vi "Sim_Control.vi"() -> ()   [LabVIEW 2009]
uses:
  <vilib>/addons/control/pid/pid.llb/PID (DBL).vi
  <vilib>/addons/control/pid/NI_PID_pid.lvlib
panel:
  out "desired turn rate and actual":cluster{"output":dbl, "Turn Rate Current":dbl}(graph)={"output"=0.0, "Turn Rate Current"=-0.0757104347794666}
  out "desired turn rate":dbl format="%.2f"
  in  "Overshoot Limit":dbl=10.0
  out "Turn Rate Current":dbl=2.609190335718722
  in  "stop":bool
  in  "Add 180":bool
  in  "Add 90":bool
  in  "Add 45":bool
  in  "Heading vs turn rate gains":T1={"proportional gain (Kc)"=-1.0, "integral time (Ti, min)"=0.0, "derivative time (Td, min)"=25.0} {"derivative time (Td, min)" format="%.5f"; "integral time (Ti, min)" format="%.5f"; "proportional gain (Kc)" format="%.5f"}
  in  "heading\ndeadband":dbl=2.0
  in  "Turn rate Control Loop":bool=TRUE
  out "Straight Voltages":cluster{"Left Voltage":dbl, "Right Voltage":dbl}
  out "Turning Voltages":cluster{"Left Voltage":dbl, "Right Voltage":dbl}={"Left Voltage"=2.5, "Right Voltage"=2.5}
  in  "Tab Control":enum32{"Sim", "Heading", "GPS"}(tab)=enum."Heading"
  out "XY Graph":T2(graph)
  out "Theta":dbl
  out "Display Heading":dbl
  in  "Initial Paremeters":T3
  out "Output Telemetry":T3
  out "Waveform Chart":T3(graph)
  in  "Iterations?":bool
  in  "Motor Voltages":cluster{"Left Voltage":dbl, "Right Voltage":dbl}={"Left Voltage"=5.0, "Right Voltage"=5.0}
  in  "Iterations":i32=300
  in  "Enable Step?":bool
  in  "step":bool
  out "Motors":cluster{"Left Voltage":dbl, "Right Voltage":dbl}(graph)
  out "Heading Error":cluster{dbl, "y":dbl, "y":dbl, "y":dbl}(graph)
  in  "Heading PID gains":T1={"proportional gain (Kc)"=0.2, "integral time (Ti, min)"=0.0, "derivative time (Td, min)"=10.0} {"derivative time (Td, min)" format="%.5f"; "integral time (Ti, min)" format="%.5f"; "proportional gain (Kc)" format="%.5f"}
  in  "Heading Control Loop?":bool=TRUE
  out "Compass Heading":dbl=1.0
  in  "Desired Heading":dbl
  out "Heading Chart":dbl(graph)
  in  "Compass Error (deg)":dbl=0.3
  in  "Compass Update Rate (hz)":dbl=8.0
  out "Longitude Chart":cluster{dbl, dbl, "Y":dbl}(graph)
  in  "GPS Update Rate (hz)":dbl=20.0
  in  "Latitude Error (m N)":dbl=1.3
  in  "Longitude Error (m E)":dbl=1.5
  out "Latitude":dbl=1.0
  out "Longitude":dbl=1.0
  out "Latitude Chart":cluster{dbl, dbl, "X":dbl}(graph)
  in  "Navigation Control Loop?":bool=TRUE
  out "Location Graph":T2(graph)
  in  "Deisired Latitude":dbl
  in  "Deisired Longitude":dbl
  out "distance to waypoint":dbl
  out "waypoint vector heading":dbl
  out "Averaged Latitude":dbl=1.0
  out "Averaged Longitude":dbl=1.0
  in  "GPS Averaging Samples":dbl=20.0
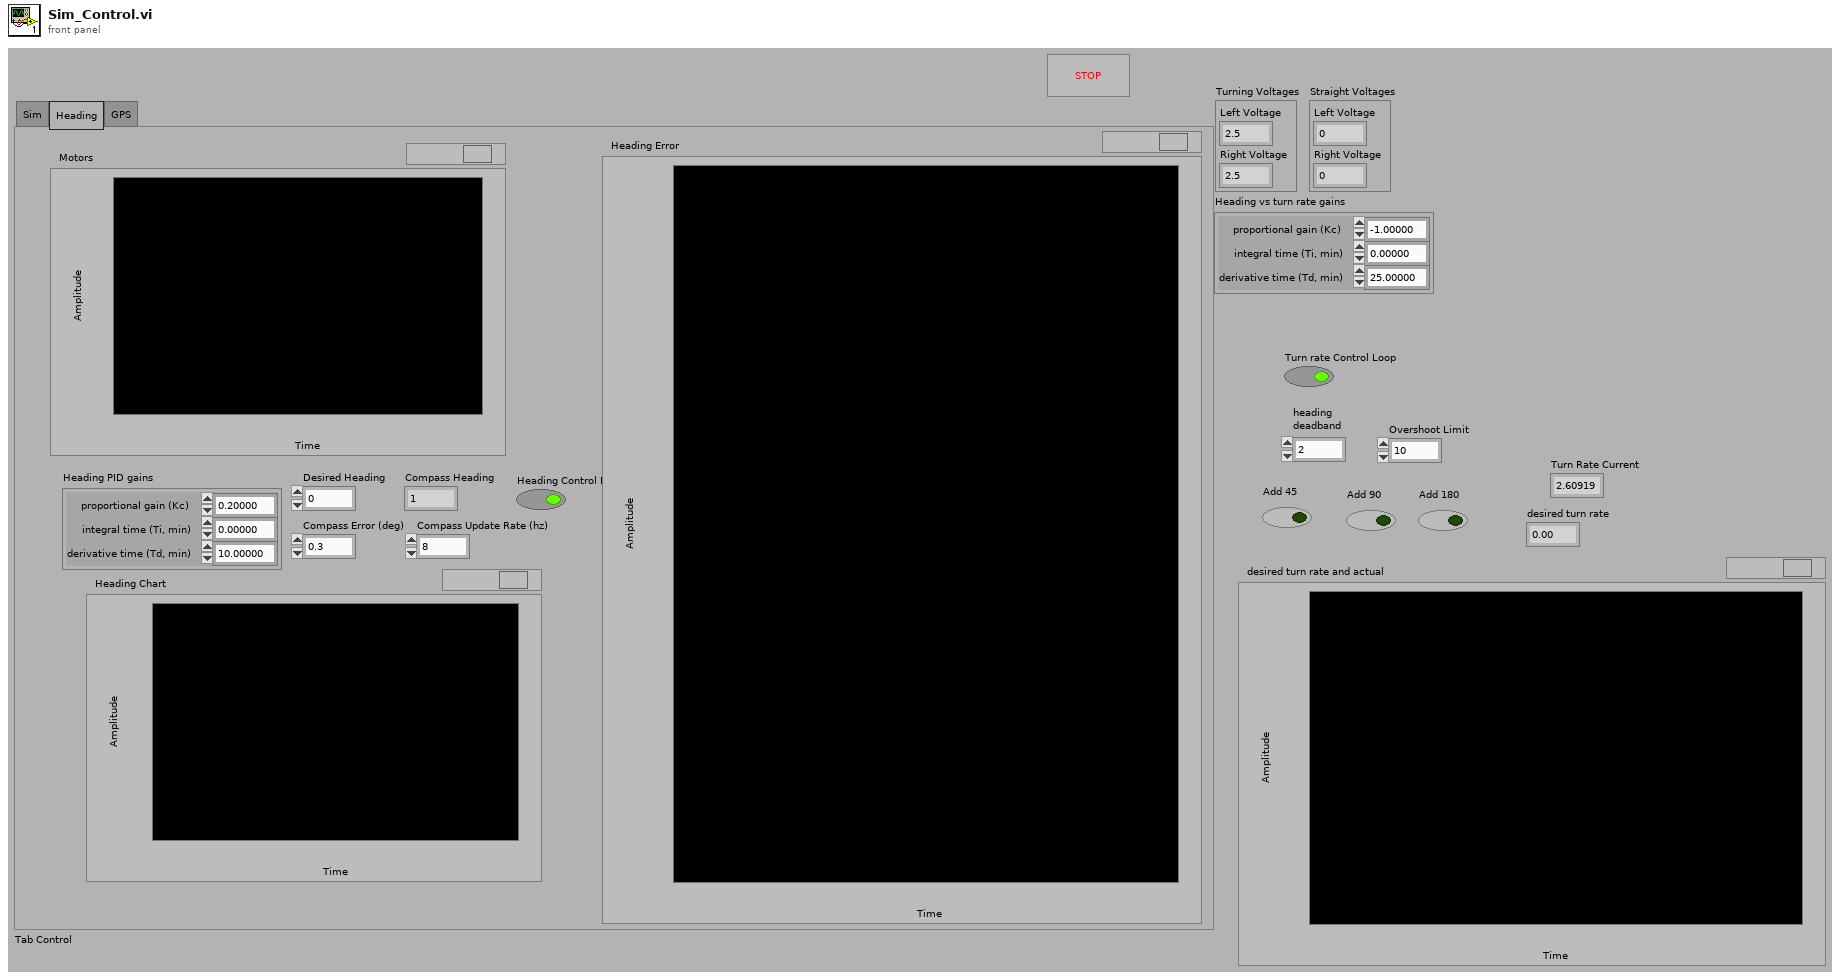
[diagram p1: front panel]
types:
  T1 = cluster{"proportional gain (Kc)":dbl, "integral time (Ti, min)":dbl, "derivative time (Td, min)":dbl}
  T2 = cluster{"initialized array":dbl[], "initialized array":dbl[]}[]
  T3 = cluster{"X":dbl, "Vx":dbl, "Ax":dbl, "Y":dbl, "Vy":dbl, "Ay":dbl, "Theta":dbl, "Omega":dbl, "Alpha":dbl}
  T4 = cluster{"X":dbl, "Vx":dbl, "Ax":dbl, "Y":dbl, "Vy":dbl, "Ay":dbl, "Theta":dbl, "Omega":dbl, "Alpha":dbl}[]
  T5 = cluster{dbl, "y":dbl, "Overshoot Limit":dbl, dbl}
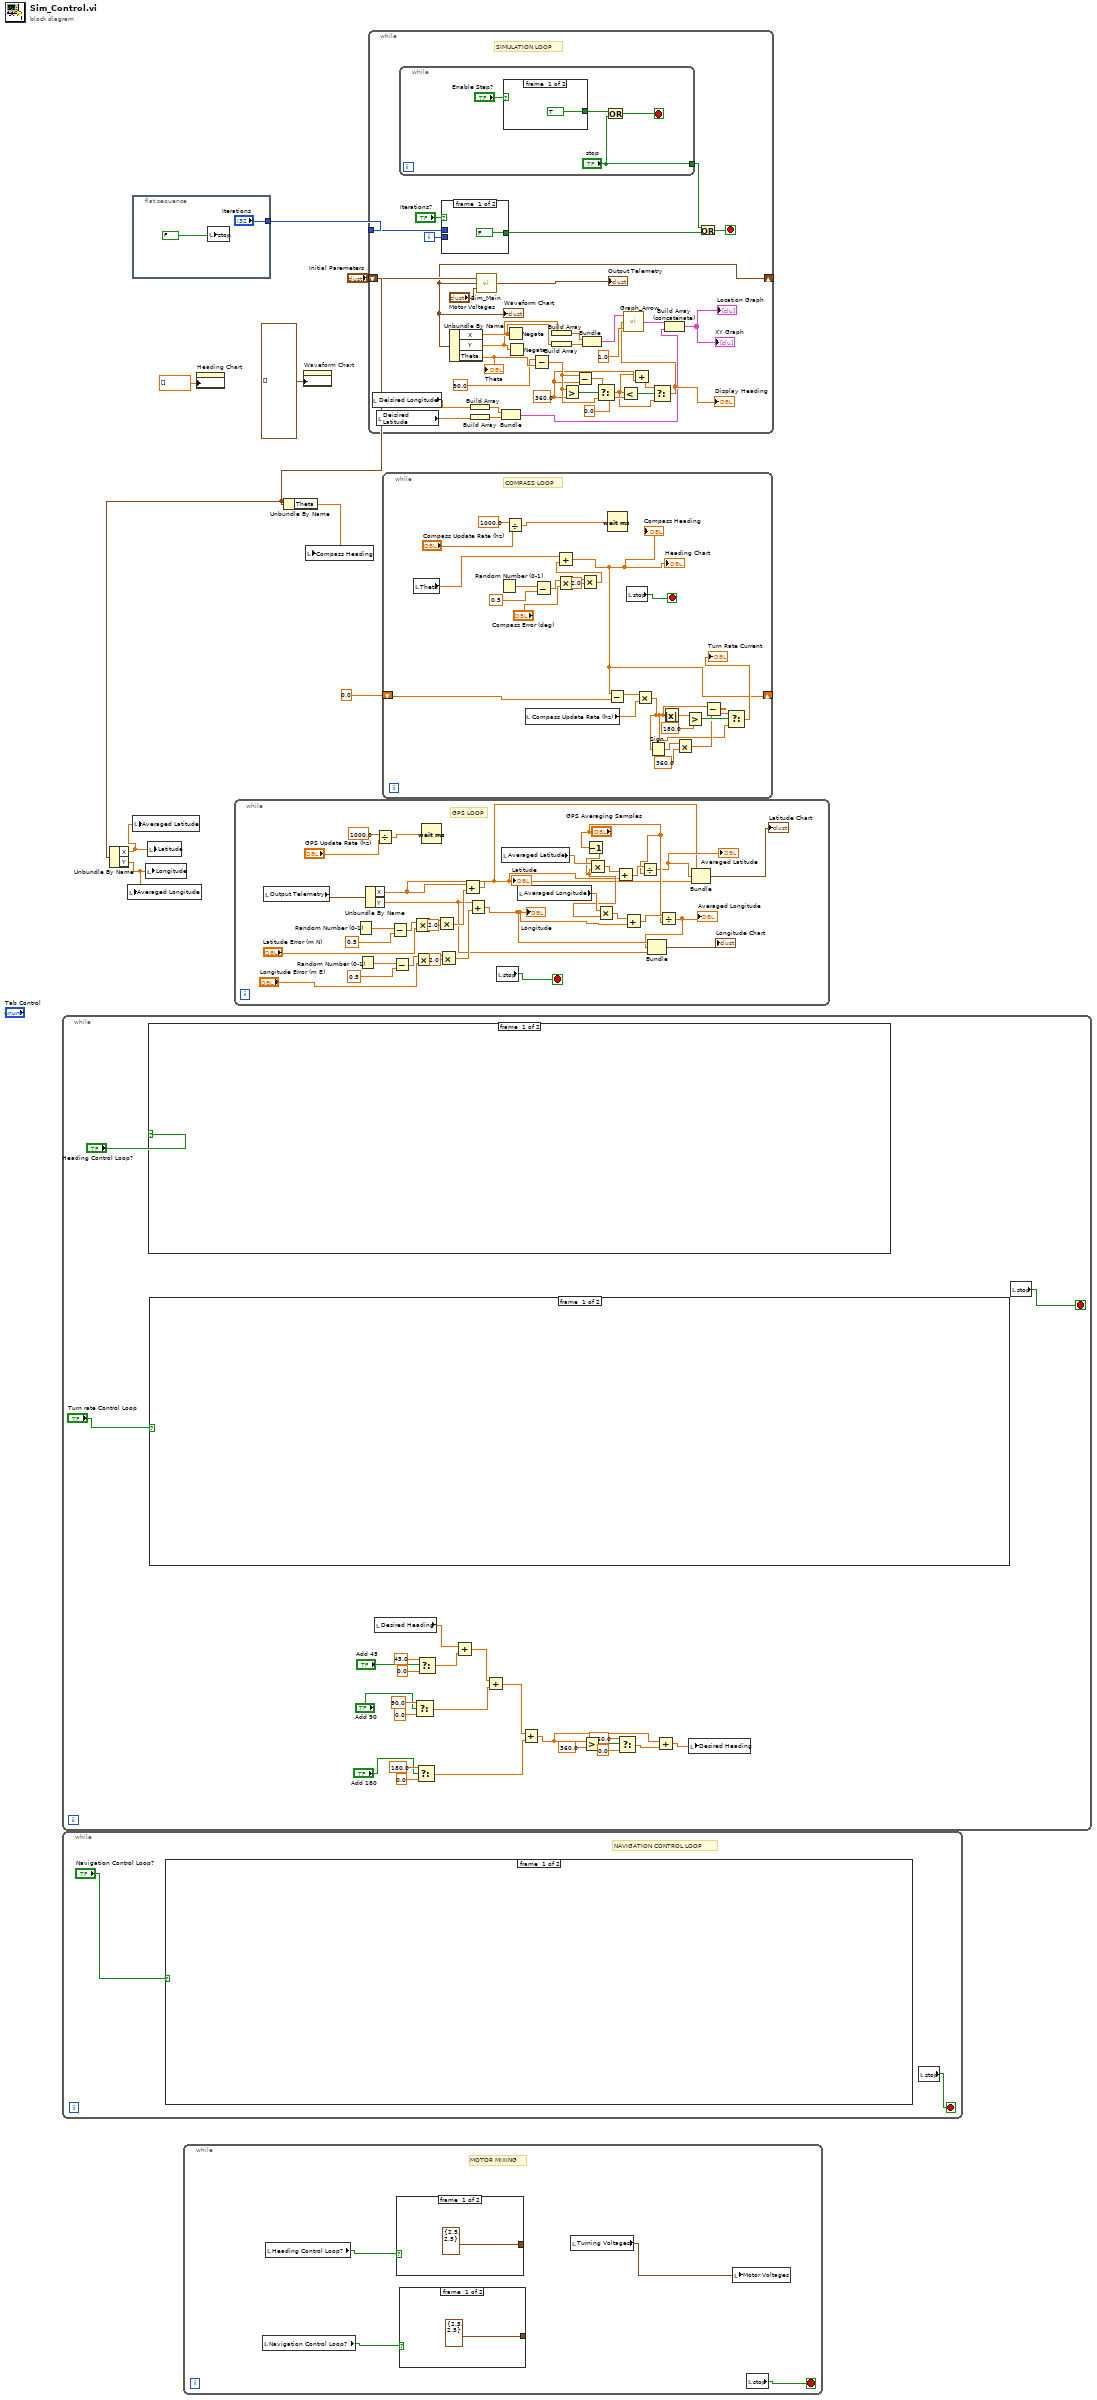
[diagram p0: block diagram]
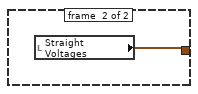
[diagram p2: hidden frame]
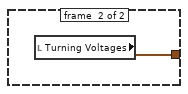
[diagram p3: hidden frame]
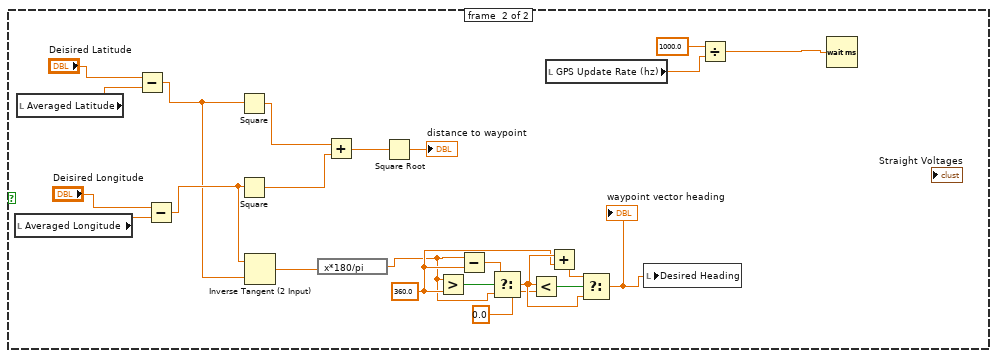
[diagram p4: hidden frame]
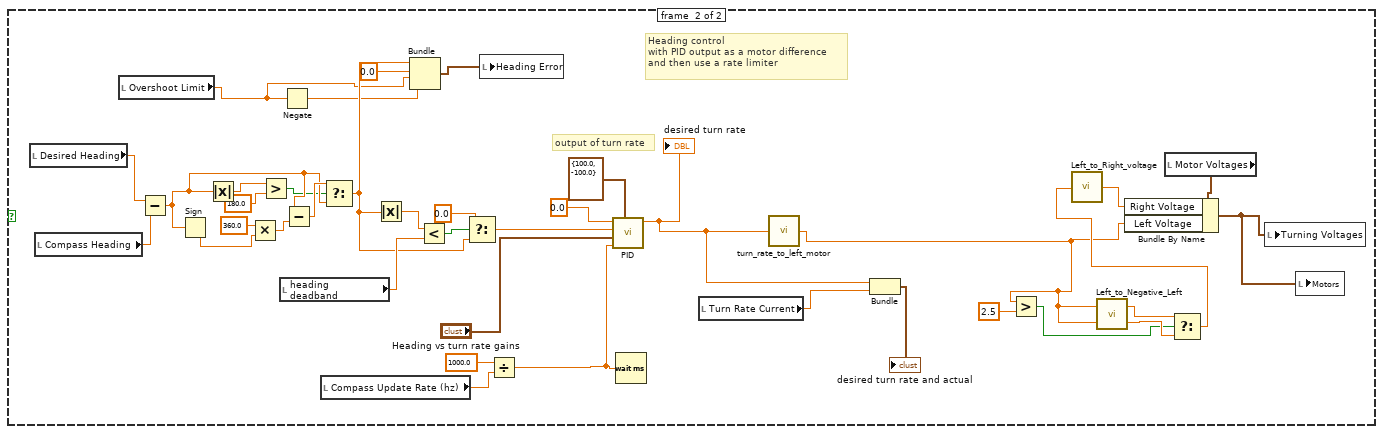
[diagram p5: hidden frame]
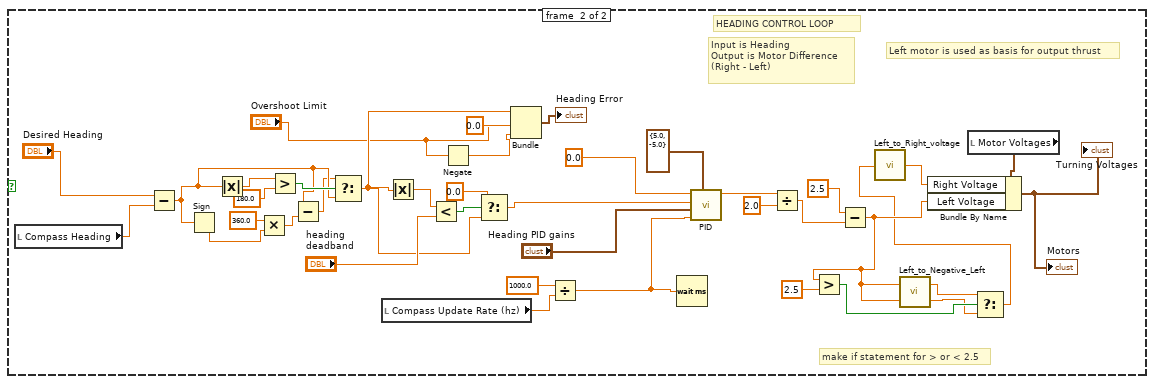
[diagram p6: hidden frame]
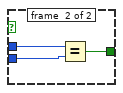
[diagram p7: hidden frame]
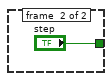
[diagram p8: hidden frame]
diagram:
  n1 = while {
    stop <- w33 stop-if-true
    n2 = case shown="True" "Heading Control Loop?" {
      frame #0 {
      }
      frame #1 {
        # "make if statement for > or < 2.5"
        # "Left motor is used as basis for output thrust"
        # "Input is Heading\nOutput is Motor Difference\n(Right - Left)"
        # "HEADING CONTROL LOOP"
        n3 = local read "Compass Heading"() -> (w100:dbl)
        n4 = Subtract(x="Desired Heading", y=w100) -> (x-y=w93:dbl)
        n5 = Sign(1:w93) -> (0:w97:dbl)
        n6 = Absolute Value(x=w93) -> (abs(x)=w98:dbl)
        n7 = Multiply(x=360.0, y=w97) -> (x*y=w92:dbl)
        n8 = Greater?(x=w98, y=180.0) -> (0:w95:bool)
        n9 = Subtract(x=w93, y=w92) -> (x-y=w91:dbl)
        n10 = Select(t=w91, s=w95, f=w93) -> (s? t:f=w76:dbl)
        n11 = local read "Compass Update Rate (hz)"() -> (w106:dbl)
        n12 = Absolute Value(x=w76) -> (abs(x)=w79:dbl)
        n13 = Less?(x=w79, y="heading\ndeadband") -> (x < y?=w78:bool)
        n14 = Negate(x="Overshoot Limit") -> (-x=w73:dbl)
        n15 = Select(t=0.0, s=w78, f=w76) -> (s? t:f=w75:dbl)
        n16 = Bundle(w76, "y"=0.0, "Overshoot Limit"="Overshoot Limit", w73) -> (→"Heading Error":T5)  [unwired: 1 in]
        n17 = Divide(x=1000.0, y=w106) -> (x/y=w90:dbl)
        n18 = Wait (ms)(milliseconds to wait=w90) -> ()  [unwired: 1 out]
        n19 = call-poly <vilib>:"PID.vi"("output range"=cluster{"output high":dbl, "output low":dbl} {"output high"=5.0, "output low"=-5.0}, "dt (s)"=w90, "PID gains"="Heading PID gains", "process variable"=w75, "setpoint"=0.0) -> ("output"=w105:dbl)  [unwired: 1 in, 5 out]
        n20 = Divide(x=w105, y=2.0) -> (x/y=w102:dbl)
        n21 = Subtract(x=2.5 ("y"), y=w102) -> (x-y=w86:dbl)
        n22 = Greater?(x=w86, y=2.5) -> (0:w85:bool)
        n23 = call "Left_to_Negative_Left.vi"("negative left in"=w86, "positive left in"=w86) -> ("positive left out"=w83:dbl, "negative left out"=w84:dbl)
        n24 = local read "Motor Voltages"() -> (w110:cluster{"Left Voltage":dbl, "Right Voltage":dbl})
        n25 = Select(t=w84, s=w85, f=w83) -> (s? t:f=w82:dbl)
        n26 = call "Left_to_Right_voltage.vi"("left"=w82) -> ("right"=w81:dbl)
        n27 = Bundle By Name(cluster=w110, "Right Voltage"=w81, "Left Voltage"=w86) -> (→"Motors" →"Turning Voltages":cluster{"Left Voltage":dbl, "Right Voltage":dbl})
      }
    }
    n28 = case shown="True" "Turn rate Control Loop" {
      frame #0 {
      }
      frame #1 {
        # "output of turn rate"
        # "Heading control\nwith PID output as a motor difference\nand then use a rate limiter"
        n29 = local read "Desired Heading"() -> (w63:dbl)
        n30 = local read "Compass Heading"() -> (w62:dbl)
        n31 = local read "Overshoot Limit"() -> (w41:dbl)
        n32 = Subtract(x=w63, y=w62) -> (x-y=w69:dbl)
        n33 = Sign(1:w69) -> (0:w65:dbl)
        n34 = Absolute Value(x=w69) -> (abs(x)=w64:dbl)
        n35 = Multiply(x=360.0, y=w65) -> (x*y=w70:dbl)
        n36 = Greater?(x=w64, y=180.0) -> (0:w67:bool)
        n37 = local read "heading\ndeadband"() -> (w57:dbl)
        n38 = Negate(x=w41) -> (-x=w40:dbl)
        n39 = Subtract(x=w69, y=w70) -> (x-y=w71:dbl)
        n40 = local read "Compass Update Rate (hz)"() -> (w55:dbl)
        n41 = Select(t=w71, s=w67, f=w69) -> (s? t:f=w56:dbl)
        n42 = Absolute Value(x=w56) -> (abs(x)=w58:dbl)
        n43 = Bundle(w56, "y"=0.0, "Overshoot Limit"=w41, w40) -> (w39:T5)  [unwired: 1 in]
        n44 = Less?(x=w58, y=w57) -> (x < y?=w59:bool)
        n45 = Select(t=0.0, s=w59, f=w56) -> (s? t:f=w42:dbl)
        n46 = local write "Heading Error"(w39) -> ()
        n47 = Divide(x=1000.0, y=w55) -> (x/y=w38:dbl)
        n48 = call-poly <vilib>:"PID.vi"("output range"=cluster{"output high":dbl, "output low":dbl} {"output high"=100.0, "output low"=-100.0}, "dt (s)"=w38, "PID gains"="Heading vs turn rate gains", "process variable"=w42, "setpoint"=0.0) -> ("output"=w37:dbl)  [unwired: 5 in, 1 out]
        "desired turn rate" <- w37
        n49 = Wait (ms)(milliseconds to wait=w38) -> ()  [unwired: 1 out]
        n50 = local read "Turn Rate Current"() -> (w36:dbl)
        n51 = call "turn_rate_to_left_motor.vi"("Turn Rate"=w37) -> ("Left Voltage"=w34:dbl)
        n52 = Bundle("output"=w37, "Turn Rate Current"=w36) -> (→"desired turn rate and actual":cluster{"output":dbl, "Turn Rate Current":dbl})  [unwired: 1 in]
        n53 = Greater?(x=w34, y=2.5) -> (0:w46:bool)
        n54 = call "Left_to_Negative_Left.vi"("negative left in"=w34, "positive left in"=w34) -> ("positive left out"=w48:dbl, "negative left out"=w47:dbl)
        n55 = local read "Motor Voltages"() -> (w44:cluster{"Left Voltage":dbl, "Right Voltage":dbl})
        n56 = Select(t=w47, s=w46, f=w48) -> (s? t:f=w49:dbl)
        n57 = call "Left_to_Right_voltage.vi"("left"=w49) -> ("right"=w50:dbl)
        n58 = Bundle By Name(cluster=w44, "Right Voltage"=w50, "Left Voltage"=w34) -> (w43:cluster{"Left Voltage":dbl, "Right Voltage":dbl})
        n59 = local write "Turning Voltages"(w43) -> ()
        n60 = local write "Motors"(w43) -> ()
      }
    }
    n61 = local read "Desired Heading"() -> (w21:dbl)
    n62 = Select(t=90.0, s="Add 90", f=0.0) -> (s? t:f=w19:dbl)
    n63 = Select(t=180.0, s="Add 180", f=0.0) -> (s? t:f=w16:dbl)
    n64 = Select(t=45.0, s="Add 45", f=0.0) -> (s? t:f=w20:dbl)
    n65 = Add(x=w21, y=w20) -> (x+y=w18:dbl)
    n66 = Add(x=w18, y=w19) -> (x+y=w17:dbl)
    n67 = Add(x=w17, y=w16) -> (x+y=w12:dbl)
    n68 = Greater?(x=w12, y=360.0) -> (0:w14:bool)
    n69 = Select(t=-360.0, s=w14, f=0.0) -> (s? t:f=w10:dbl)
    n70 = Add(x=w12, y=w10) -> (x+y=w13:dbl)
    n71 = local write "Desired Heading"(w13) -> ()
    n72 = local read "stop"() -> (w33:bool)
  }
  n73 = while {
    stop <- w111 stop-if-true
    # "NAVIGATION CONTROL LOOP"
    n74 = case shown="True" "Navigation Control Loop?" {
      frame #0 {
      }
      frame #1 {
        w122 = 360.0 ("y")
        n75 = local read "Averaged Longitude"() -> (w132:dbl)
        n76 = local read "Averaged Latitude"() -> (w134:dbl)
        n77 = Subtract(x="Deisired Latitude", y=w134) -> (x-y=w125:dbl)
        n78 = Subtract(x="Deisired Longitude", y=w132) -> (x-y=w126:dbl)
        n79 = Square(x=w125) -> (x^2=w130:dbl)
        n80 = Square(x=w126) -> (x^2=w129:dbl)
        n81 = Inverse Tangent (2 Input)(1:w125, 2:w126) -> (0:w127:dbl)
        n82 = expression code="x*180/pi"(w127) -> (w117:dbl)
        n83 = Add(x=w130, y=w129) -> (x+y=w131:dbl)
        n84 = Square Root(x=w131) -> (sqrt(x)=→"distance to waypoint":dbl)
        n85 = Greater?(x=w117, y=w122) -> (0:w118:bool)
        n86 = Subtract(x=w117, y=w122) -> (x-y=w119:dbl)
        n87 = Select(t=w119, s=w118, f=w117) -> (s? t:f=w124:dbl)
        n88 = Less?(x=w124, y=0.0) -> (x < y?=w121:bool)
        n89 = local read "GPS Update Rate (hz)"() -> (w114:dbl)
        n90 = Add(x=w124, y=w122) -> (x+y=w123:dbl)
        n91 = Select(t=w123, s=w121, f=w124) -> (s? t:f=w116:dbl)
        "waypoint vector heading" <- w116
        n92 = local write "Desired Heading"(w116) -> ()
        n93 = Divide(x=1000.0, y=w114) -> (x/y=w115:dbl)
        n94 = Wait (ms)(milliseconds to wait=w115) -> ()  [unwired: 1 out]
      }
    }
    n95 = local read "stop"() -> (w111:bool)
  }
  n96 = Unbundle By Name("Initial Paremeters") -> ("X"=w2:dbl, "Y"=w3:dbl)
  n97 = local write "Averaged Longitude"(w3) -> ()
  n98 = local write "Averaged Latitude"(w2) -> ()
  n99 = flat-sequence {
    tunnel: ["Iterations"] -> w7
    frame #0 {
      n100 = local write "stop"(FALSE) -> ()
    }
  }
  n101 = local write "Longitude"(w3) -> ()
  n102 = local write "Latitude"(w2) -> ()
  n103 = while {
    stop <- w139 stop-if-true
    # "MOTOR MIXING"
    n104 = local read "Navigation Control Loop?"() -> (w140:bool)
    n105 = local read "Heading Control Loop?"() -> (w141:bool)
    n106 = case shown="True" w141 {
      tunnel: [cluster{"Left Voltage":dbl, "Right Voltage":dbl} {"Left Voltage"=2.5, "Right Voltage"=2.5} ("Turning Voltages") w145] -> _
      frame #0 {
      }
      frame #1 {
        n107 = local read "Turning Voltages"() -> (w145:cluster{"Left Voltage":dbl, "Right Voltage":dbl})
      }
    }
    n108 = case shown="True" w140 {
      tunnel: [cluster{"Left Voltage":dbl, "Right Voltage":dbl} {"Left Voltage"=2.5, "Right Voltage"=2.5} ("Turning Voltages") w143] -> _
      frame #0 {
      }
      frame #1 {
        n109 = local read "Straight Voltages"() -> (w143:cluster{"Left Voltage":dbl, "Right Voltage":dbl})
      }
    }
    n110 = local read "Turning Voltages"() -> (w138:cluster{"Left Voltage":dbl, "Right Voltage":dbl})
    n111 = local write "Motor Voltages"(w138) -> ()
    n112 = local read "stop"() -> (w139:bool)
  }
  n113 = property on="Heading Chart" class="WFChart (strict)"("History Data"=dbl[] []) -> ()  [unwired: 2 in, 2 out]
  n114 = while {
    stop <- w180 stop-if-true
    # "GPS LOOP"
    n115 = local read "Output Telemetry"() -> (w179:T3)
    n116 = Random Number (0-1)() -> (number: 0 to 1=w172:dbl)
    n117 = Random Number (0-1)() -> (number: 0 to 1=w171:dbl)
    n118 = Unbundle By Name(w179) -> ("X"=w147:dbl, "Y"=w146:dbl)
    n119 = Divide(x=1000.0, y="GPS Update Rate (hz)") -> (x/y=w178:dbl)
    n120 = Subtract(x=w172, y=0.5) -> (x-y=w173:dbl)
    n121 = Subtract(x=w171, y=0.5) -> (x-y=w170:dbl)
    n122 = Multiply(x=w173, y="Latitude Error (m N)") -> (x*y=w174:dbl)
    n123 = Multiply(x=w170, y="Longitude Error (m E)") -> (x*y=w169:dbl)
    n124 = Wait (ms)(milliseconds to wait=w178) -> ()  [unwired: 1 out]
    n125 = Multiply(x=w174, y=2.0) -> (x*y=w162:dbl)
    n126 = Multiply(x=w169, y=2.0) -> (x*y=w163:dbl)
    n127 = Add(x=w147, y=w162) -> (x+y=w148:dbl)
    "Latitude" <- w148
    n128 = Add(x=w146, y=w163) -> (x+y=w156:dbl)
    "Longitude" <- w156
    n129 = local read "stop"() -> (w180:bool)
    n130 = local read "Averaged Latitude"() -> (w160:dbl)
    n131 = local read "Averaged Longitude"() -> (w158:dbl)
    n132 = Decrement(x="GPS Averaging Samples") -> (x-1=w157:dbl)
    n133 = Multiply(x=w160, y=w157) -> (x*y=w161:dbl)
    n134 = Multiply(x=w158, y=w157) -> (x*y=w159:dbl)
    n135 = Add(x=w161, y=w148) -> (x+y=w155:dbl)
    n136 = Add(x=w159, y=w156) -> (x+y=w154:dbl)
    n137 = Divide(x=w155, y="GPS Averaging Samples") -> (x/y=w150:dbl)
    "Averaged Latitude" <- w150
    n138 = Divide(x=w154, y="GPS Averaging Samples") -> (x/y=w152:dbl)
    "Averaged Longitude" <- w152
    n139 = Bundle(w156, w152, "Y"=w146) -> (→"Longitude Chart":cluster{dbl, dbl, "Y":dbl})  [unwired: 1 in]
    n140 = Bundle(w148, w150, "X"=w147) -> (→"Latitude Chart":cluster{dbl, dbl, "X":dbl})  [unwired: 1 in]
  }
  n141 = Unbundle By Name("Initial Paremeters") -> ("Theta"=w6:dbl)
  n142 = property on="Waveform Chart" class="WFChart (strict)"("History Data"=T4 []) -> ()  [unwired: 2 in, 2 out]
  n143 = local write "Compass Heading"(w6) -> ()
  n144 = while {
    shift-right: [w211] -> _
    shift-left: "Initial Paremeters" -> [w213]
    tunnel: w7 -> [w204]
    i -> [w206]
    stop <- w207 stop-if-true
    w191 = 360.0 ("y")
    # "SIMULATION LOOP"
    n145 = local read "Deisired Longitude"() -> (w182:dbl)
    n146 = local read "Deisired Latitude"() -> (w181:dbl)
    n147 = while {
      tunnel: ["stop"] -> w208
      stop <- w220 stop-if-true
      n148 = case shown="True" "Enable Step?" {
        tunnel: [TRUE ("step") "step"] -> w221
        frame #0 {
        }
        frame #1 {
        }
      }
      n149 = Or(x=w221, y="stop") -> (x .or. y?=w220:bool)
    }
    n150 = case shown="False" "Iterations?" {
      tunnel: w206 -> [_ w217]
      tunnel: [FALSE w216] -> w205
      tunnel: w204 -> [_ w215]
      frame #0 {
      }
      frame #1 {
        n151 = Equal?(x=w215, y=w217) -> (x = y?=w216:bool)
      }
    }
    n152 = Build Array(w182) -> (w184:dbl[])
    n153 = Build Array(w181) -> (w185:dbl[])
    n154 = call "Sim_Main.vi"("Motor Voltages"="Motor Voltages", "Input Telemetry"=w213) -> ("Output Telemetry"=w211:T3)
    "Waveform Chart" <- w211
    "Output Telemetry" <- w211
    n155 = Unbundle By Name(w211) -> ("X"=w201:dbl, "Y"=w200:dbl, "Theta"=w199:dbl)
    "Theta" <- w199
    n156 = Bundle(w184, w185) -> (w183:cluster{dbl[], dbl[]})  [unwired: 1 in]
    n157 = Negate(x=w201) -> ()  [unwired: 1 out]
    n158 = Negate(x=w200) -> ()  [unwired: 1 out]
    n159 = Subtract(x=90.0, y=w199) -> (x-y=w195:dbl)
    n160 = Build Array(w200) -> (w210:dbl[])
    n161 = Build Array(w201) -> (w209:dbl[])
    n162 = Greater?(x=w195, y=w191) -> (0:w197:bool)
    n163 = Subtract(x=w195, y=w191) -> (x-y=w196:dbl)
    n164 = Bundle(w210, w209) -> (w202:cluster{dbl[], dbl[]})  [unwired: 1 in]
    n165 = Select(t=w196, s=w197, f=w195) -> (s? t:f=w189:dbl)
    n166 = Less?(x=w189, y=0.0) -> (x < y?=w193:bool)
    n167 = Add(x=w189, y=w191) -> (x+y=w190:dbl)
    n168 = Select(t=w190, s=w193, f=w189) -> (s? t:f=w188:dbl)
    "Display Heading" <- w188
    n169 = call "Graph_Arrow.vi"("magnitude"=1.0, "Heading"=w188, "plot data"=w202) -> ("XY Graph"=w187:T2)
    n170 = Build Array (concatenate)(w187, w183) -> (→"XY Graph" →"Location Graph":T2)
    n171 = Or(x=w208, y=w205) -> (x .or. y?=w207:bool)
  }
  n172 = while {
    shift-right: [w224] -> _
    shift-left: 0.0 ("y") -> [w236]
    stop <- w246 stop-if-true
    # "COMPASS LOOP"
    n173 = local read "Theta"() -> (w238:dbl)
    n174 = Random Number (0-1)() -> (number: 0 to 1=w245:dbl)
    n175 = Divide(x=1000.0, y="Compass Update Rate (hz)") -> (x/y=w237:dbl)
    n176 = local read "Compass Update Rate (hz)"() -> (w235:dbl)
    n177 = Subtract(x=w245, y=0.5) -> (x-y=w243:dbl)
    n178 = Multiply(x=w243, y="Compass Error (deg)") -> (x*y=w241:dbl)
    n179 = Multiply(x=w241, y=2.0) -> (x*y=w240:dbl)
    n180 = Add(x=w238, y=w240) -> (x+y=w224:dbl)
    "Compass Heading" <- w224
    "Heading Chart" <- w224
    n181 = Wait (ms)(milliseconds to wait=w237) -> ()  [unwired: 1 out]
    n182 = Subtract(x=w224, y=w236) -> (x-y=w234:dbl)
    n183 = local read "stop"() -> (w246:bool)
    n184 = Multiply(x=w234, y=w235) -> (x*y=w226:dbl)
    n185 = Sign(1:w226) -> (0:w231:dbl)
    n186 = Absolute Value(x=w226) -> (abs(x)=w233:dbl)
    n187 = Multiply(x=w231, y=360.0) -> (x*y=w228:dbl)
    n188 = Greater?(x=w233, y=180.0) -> (0:w229:bool)
    n189 = Subtract(x=w226, y=w228) -> (x-y=w227:dbl)
    n190 = Select(t=w227, s=w229, f=w226) -> (s? t:f=→"Turn Rate Current":dbl)
  }
